vi "Shutdown.vi"(8 "error in (no error)":errorcluster, 11 "Microscope in":refnum<class "Microscope.lvclass">) -> (0 "error out":errorcluster, 3 "Microscope out":refnum<class "Microscope.lvclass">)   [LabVIEW 2020, in "Microscope.lvlib" / "Microscope.lvclass"]
uses:
  Microscope.lvclass
  Microscope.lvclass/Microscope.ctl
  <vilib>/ActorFramework/Message Enqueuer/Message Enqueuer.lvclass/Message Enqueuer.ctl
  <vilib>/ActorFramework/Message Enqueuer/Enqueue.vi
  <vilib>/ActorFramework/Stop Msg/Stop Msg.lvclass
  C:/Program Files/National Instruments/LabVIEW 2020/vi.lib/ActorFramework/Message/Message.lvclass
  <vilib>/ActorFramework/Message Priority Queue/Priority Enqueue.vi
  Component/Device/Device/Device.lvclass
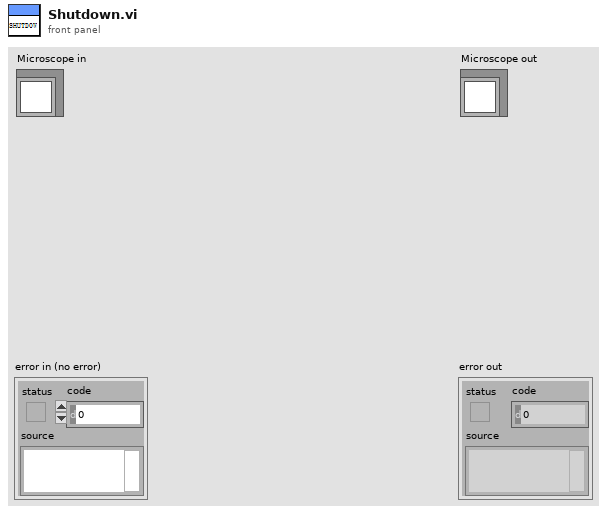
[diagram p1: front panel]
types:
  T1 = map{string, refnum<class "Message Enqueuer.lvclass">}
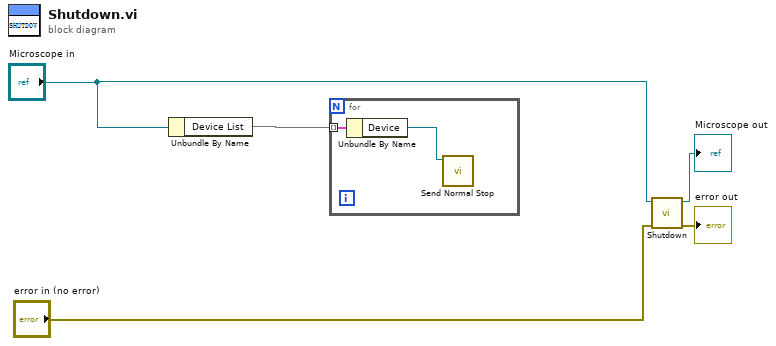
[diagram p0: block diagram]
diagram:
  n1 = Unbundle By Name("Microscope in") -> ("Device List"=w1:T1)
  n2 = for {
    tunnel: w1 -> [w7] mode=indexing
    n3 = Unbundle By Name(w7) -> ("Device"=w6:refnum<class "Message Enqueuer.lvclass">)
    n4 = call <vilib>:"Send Normal Stop.vi"("Message Enqueuer"=w6) -> ()  [unwired: 10 in, 1 out]
  }
  n5 = call-parent "Shutdown.vi"("error in (no error)"="error in (no error)", "Device in"="Microscope in") -> ("error out"=→"error out":errorcluster, "Device out"=→"Microscope out":refnum<class "Microscope.lvclass">)  [unwired: 8 in]
